vi "GyroAuto.vi"(11 "Distance(In)":dbl) -> ()   [LabVIEW 2015]
uses:
  <vilib>/addons/control/pid/pid.llb/PID (DBL).vi
  <vilib>/addons/control/pid/NI_PID_pid.lvlib
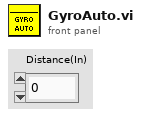
[diagram p1: front panel]
types:
  T1 = cluster{"proportional gain (Kc)":dbl, "integral time (Ti, min)":dbl, "derivative time (Td, min)":dbl}
  T2 = typedef "WPI_GyroDevRef.ctl" = cluster{"DevStatus":errorcluster, "Analog Module":T3, "Analog Channel":T4, "Offset":dbl, "Gain (VoltsPerDegree/Second)":dbl}
  T3 = typedef "FPGA_TypedefAnalogModule.ctl" = enum16{"Analog Module 1", "Analog Module 2"}
  T4 = typedef "FPGA_AIChannel.ctl" = enum8{"AI 1", "AI 2", "AI 3", "AI 4", "AI 5", "AI 6", "AI 7", "AI 8", "Invalid"}
  T5 = typedef "WPI_EncoderDevRef.ctl" = cluster{"DevStatus":errorcluster, "EncoderIndex":T6, "CounterIndex":T7, "DistancePerCount":dbl, "Decoding Type":T8}
  T6 = typedef "FPGA_EncoderIdx.ctl" = enum8{"Enc 0", "Enc 1", "Enc 2", "Enc 3", "Invalid"}
  T7 = typedef "FPGA_CounterCtrSystemIndex.ctl" = enum8{"Ctr 0", "Ctr 1", "Ctr 2", "Ctr 3", "Ctr 4", "Ctr 5", "Ctr 6", "Ctr 7", "Invalid"}
  T8 = typedef "WPI_EncoderType.ctl" = enum16{"1x", "2x", "4x"}
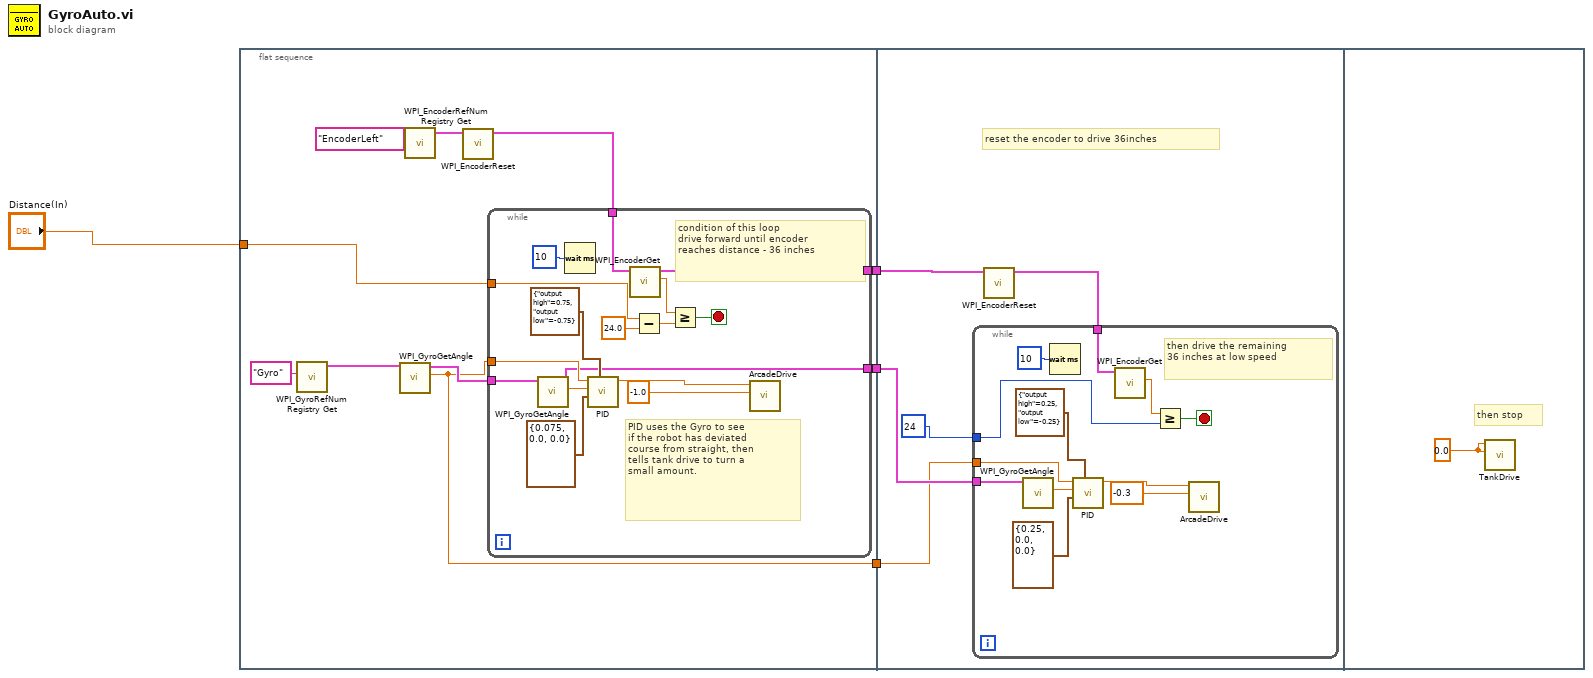
[diagram p0: block diagram]
diagram:
  n1 = flat-sequence {
    tunnel: [w12] -> w4
    tunnel: [w9] -> w3
    tunnel: [w6] -> w2
    tunnel: "Distance(In)" -> [w5]
    tunnel: w4 -> [w34]
    tunnel: w3 -> [w32]
    tunnel: w2 -> [w33]
    frame #0 {
      n2 = call <vilib>:"WPI_GyroRefNum Registry Get.vi"("refnum name"="Gyro") -> ("GyroDevRef"=w11:T2)  [unwired: 9 in, 1 out]
      n3 = call <vilib>:"WPI_GyroGetAngle.vi"("GyroDevRef"=w11) -> ("Angle"=w9:dbl, "GyroDevRef"=w10:T2)  [unwired: 7 in, 2 out]
      n4 = call <vilib>:"WPI_EncoderRefNum Registry Get.vi"("refnum name"="EncoderLeft") -> ("EncoderDevRef"=w8:T5)  [unwired: 9 in, 1 out]
      n5 = call <vilib>:"WPI_EncoderReset.vi"("EncoderDevRef"=w8) -> ("EncoderDevRef"=w7:T5)  [unwired: 9 in, 1 out]
      n6 = while {
        tunnel: w5 -> [w21]
        tunnel: w7 -> [w24]
        tunnel: [w20] -> w6
        tunnel: [w15] -> w12
        tunnel: w9 -> [w19]
        tunnel: w10 -> [w18]
        stop <- w30 stop-if-true
        # "PID uses the Gyro to see \nif the robot has deviated \ncourse from straight, then\ntells tank drive to turn a \nsmall amount."
        # "condition of this loop\ndrive forward until encoder \nreaches distance - 36 inches"
        n7 = call <vilib>:"WPI_GyroGetAngle.vi"("GyroDevRef"=w18) -> ("Angle"=w27:dbl, "GyroDevRef"=w15:T2)  [unwired: 7 in, 2 out]
        n8 = Wait (ms)(milliseconds to wait=10) -> ()  [unwired: 1 out]
        n9 = call-poly <vilib>:"PID.vi"("output range"=cluster{"output high":dbl, "output low":dbl} {"output high"=0.75, "output low"=-0.75}, "PID gains"=T1 {"proportional gain (Kc)"=0.075, "integral time (Ti, min)"=0.0, "derivative time (Td, min)"=0.0}, "process variable"=w27, "setpoint"=w19) -> ("output"=w16:dbl)  [unwired: 6 in, 1 out]
        n10 = call <vilib>:"WPI_EncoderGet.vi"("EncoderDevRef"=w24) -> ("Distance"=w26:dbl, "EncoderDevRef"=w20:T5)  [unwired: 5 in, 4 out]
        n11 = Subtract(x=w21, y=24.0) -> (x-y=w23:dbl)
        n12 = Greater Or Equal?(x=w26, y=w23) -> (x >= y?=w30:bool)
        n13 = call "ArcadeDrive.vi"("y"=-1.0, "x"=w16) -> ()  [unwired: 10 in]
      }
    }
    frame #1 {
      # "reset the encoder to drive 36inches"
      n14 = call <vilib>:"WPI_EncoderReset.vi"("EncoderDevRef"=w33) -> ("EncoderDevRef"=w35:T5)  [unwired: 9 in, 1 out]
      n15 = while {
        tunnel: 24 -> [w41]
        tunnel: w35 -> [w40]
        tunnel: w34 -> [w39]
        tunnel: w32 -> [w38]
        stop <- w47 stop-if-true
        # "then drive the remaining\n36 inches at low speed"
        n16 = call <vilib>:"WPI_GyroGetAngle.vi"("GyroDevRef"=w39) -> ("Angle"=w44:dbl)  [unwired: 7 in, 3 out]
        n17 = Wait (ms)(milliseconds to wait=10) -> ()  [unwired: 1 out]
        n18 = call-poly <vilib>:"PID.vi"("output range"=cluster{"output high":dbl, "output low":dbl} {"output high"=0.25, "output low"=-0.25}, "PID gains"=T1 {"proportional gain (Kc)"=0.25, "integral time (Ti, min)"=0.0, "derivative time (Td, min)"=0.0}, "process variable"=w44, "setpoint"=w38) -> ("output"=w36:dbl)  [unwired: 6 in, 1 out]
        n19 = call <vilib>:"WPI_EncoderGet.vi"("EncoderDevRef"=w40) -> ("Distance"=w43:dbl)  [unwired: 5 in, 5 out]
        n20 = Greater Or Equal?(x=w43, y=w41) -> (x >= y?=w47:bool)
        n21 = call "ArcadeDrive.vi"("y"=-0.3, "x"=w36) -> ()  [unwired: 10 in]
      }
    }
    frame #2 {
      w48 = 0.0 ("Left axis value")
      # "then stop"
      n22 = call "TankDrive.vi"("right"=w48, "left"=w48) -> ()  [unwired: 10 in]
    }
  }
